vi "Sender UI.vi"(11 "error in (no error)":errorcluster) -> (15 "Error Out":errorcluster)   [LabVIEW 2022 SP3, in "Sender.lvclass"]
doc: "This VI acts as a sender where user selects the data type and the transmission type to send to the receiver."
uses:
  Sender.lvclass
  Controls/Operation.ctl
  Controls/State Cluster.ctl
  Controls/Sender Data Cluster.ctl
  Controls/Communication Mode.ctl
  Communication/Communication.lvclass
  Controls/User Event Operation.ctl
  Downloads/Sample PC Template/Sample PC Template/Typedefs/Data.ctl
  Downloads/Sample PC Template/Sample PC Template/Sample PC Template.lvlib
panel:
  in  "Stop Data":bool
  in  "Transmission Type":T1=enum."Notify With Data"
  in  "Data Type":string(combo)="Numeric Data"
  in  "Send":bool
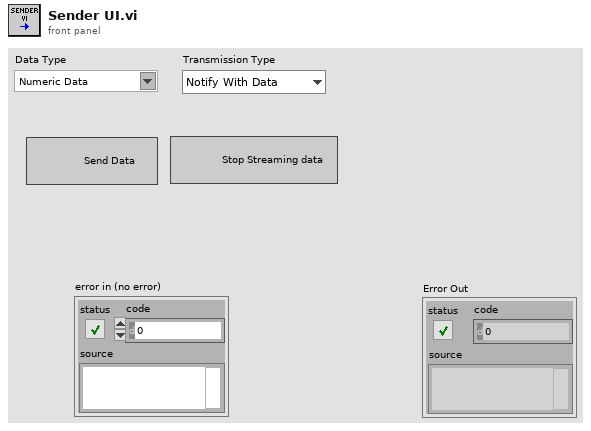
[diagram p1: front panel]
types:
  T1 = typedef "Communication Mode.ctl" = enum16{"Notify", "Notify With Data", "Stream Data"}
  T2 = typedef "User Event Operation.ctl" = enum16{"Obtain", "Generate", "Release"}
  T3 = typedef "State Cluster.ctl" = cluster{"State":string, "Data":variant}
  T4 = typedef "Operation.ctl" = enum16{"Create", "Enqueue", "Enqueue N", "Enstack", "Dequeue", "Flush", "Release"}
  T5 = enum8{"Enabled", "Disabled", "Disabled and Grayed Out"}
  T6 = typedef "Sample PC Template.lvlib/Data.ctl" = cluster{"State":string, "Data":variant}
  T7 = typedef "Sender Data Cluster.ctl" = cluster{"user event out":refnum<user-event>, "Selected Data Type":string, "Receiver VI Reference":refnum<vi>, "Transmission Type":T1, "Start Time":dbl, "Stop Stream Data":bool, "Communication Parent Class":refnum<class "Communication.lvclass">}
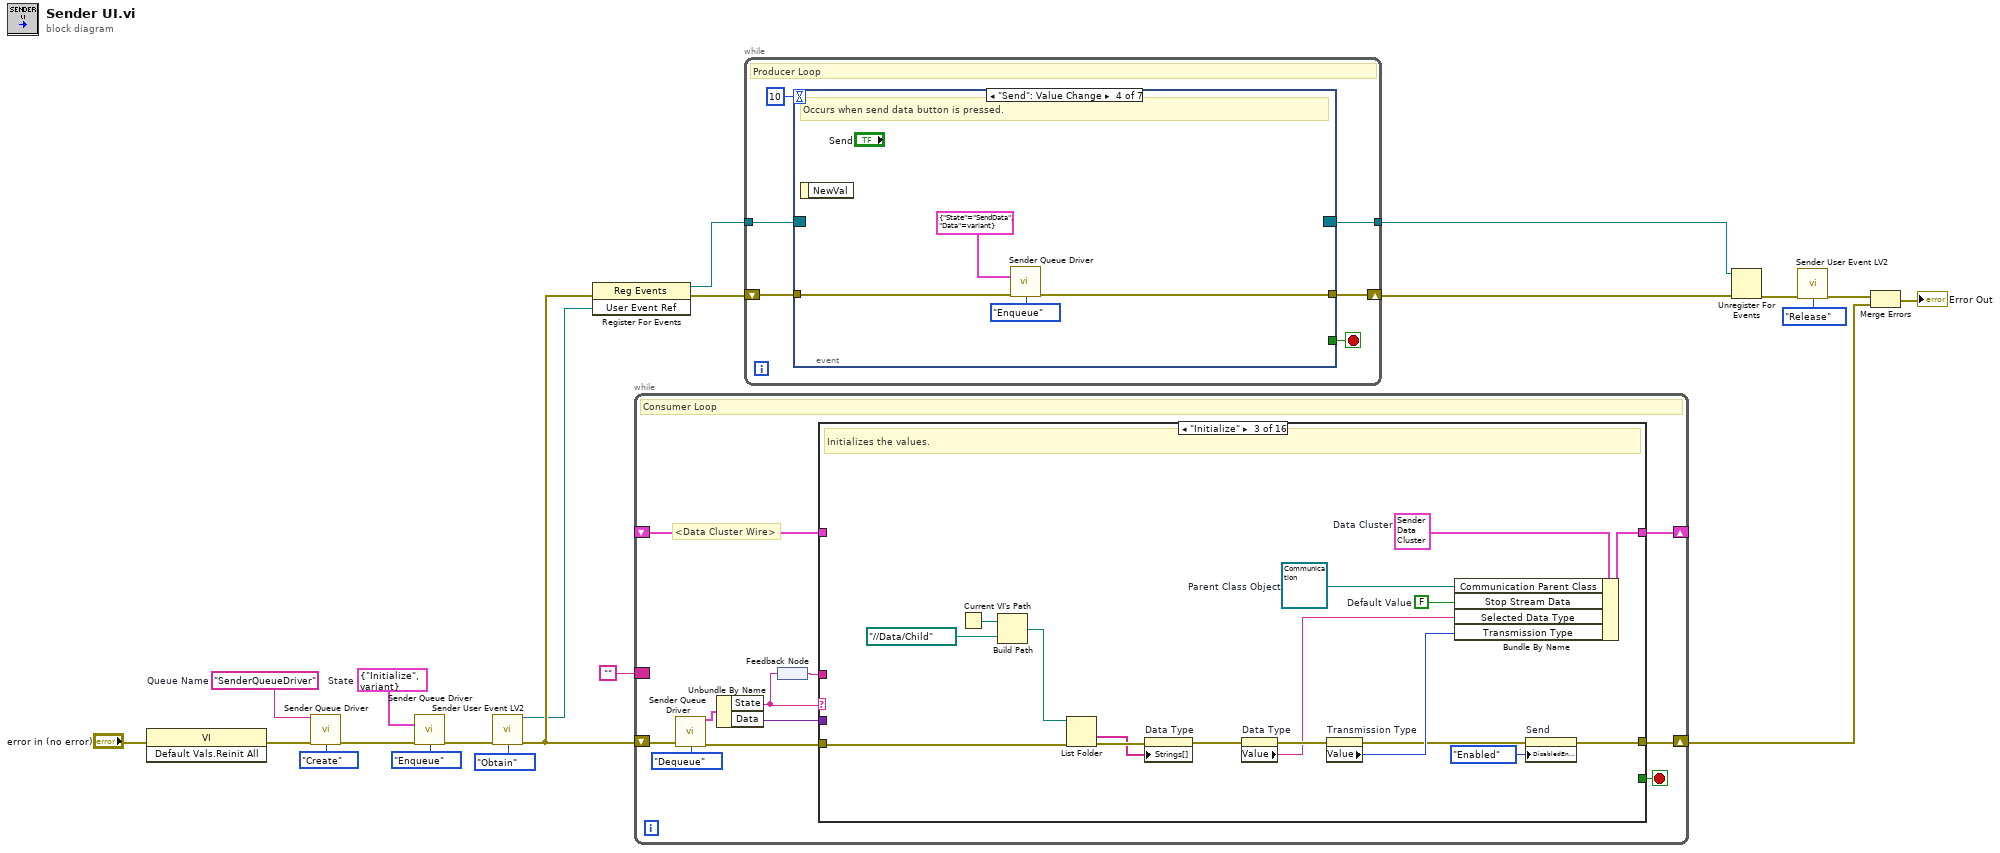
[diagram p0: block diagram]
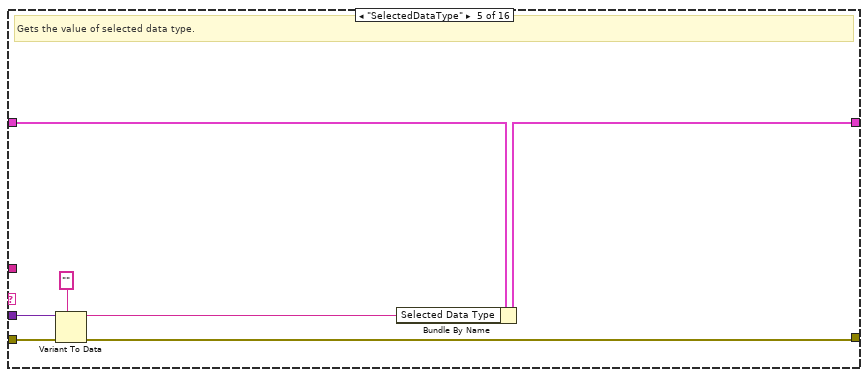
[diagram p5: hidden frame]
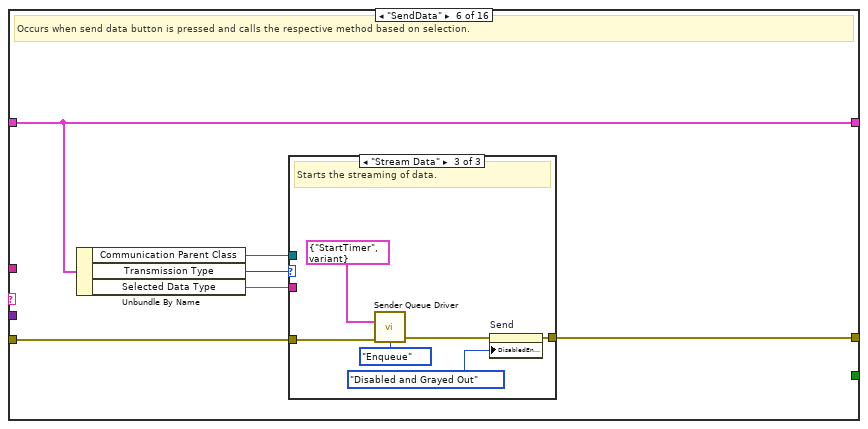
[diagram p6: hidden frame]
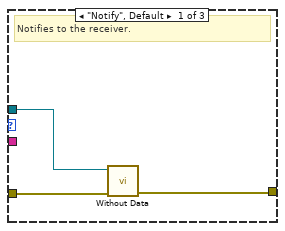
[diagram p7: hidden frame]
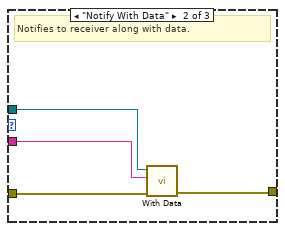
[diagram p8: hidden frame]
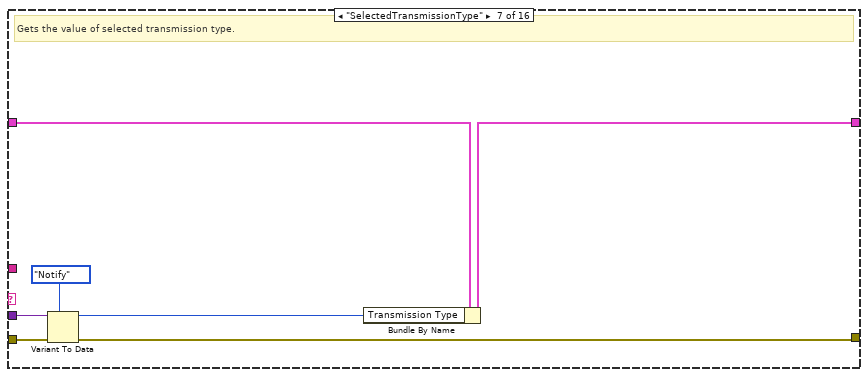
[diagram p9: hidden frame]
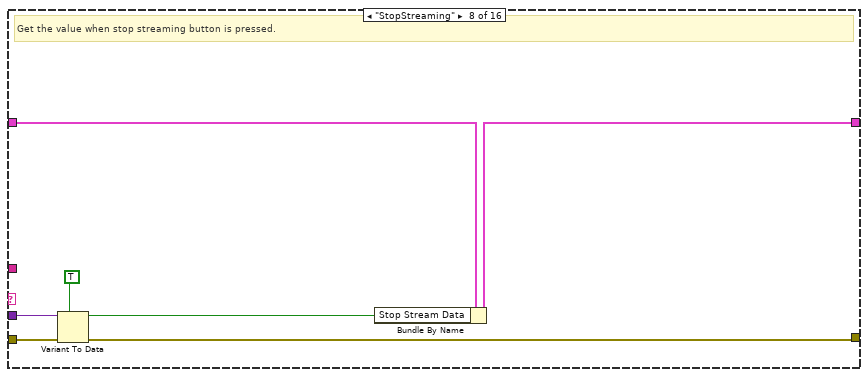
[diagram p10: hidden frame]
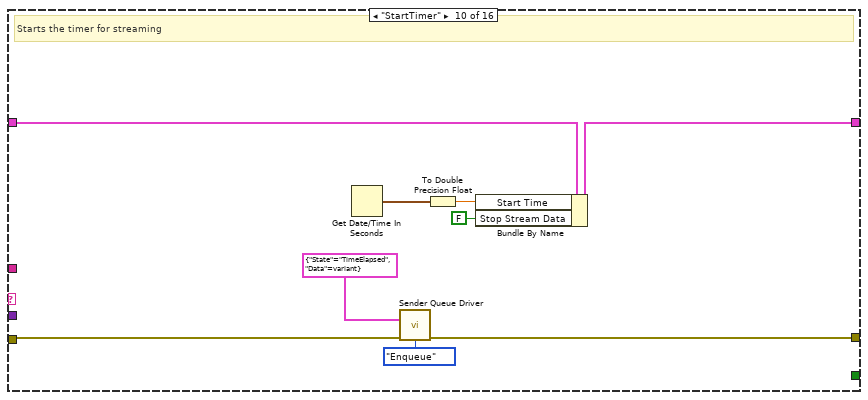
[diagram p12: hidden frame]
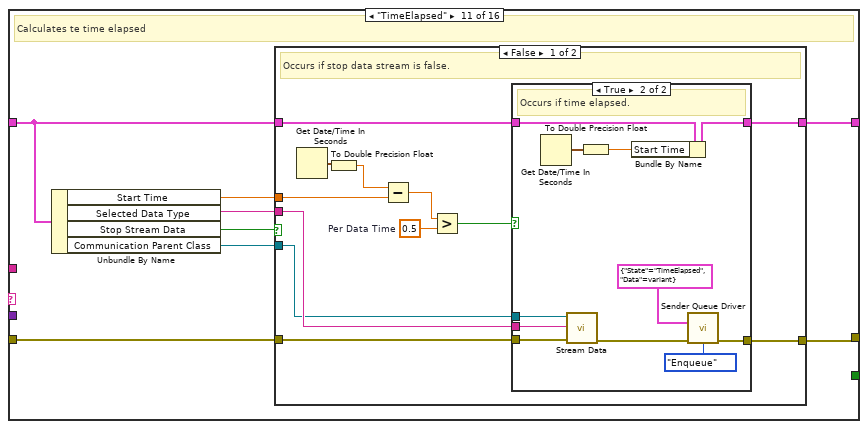
[diagram p13: hidden frame]
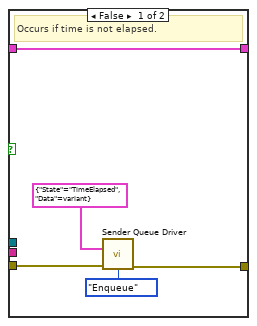
[diagram p14: hidden frame]
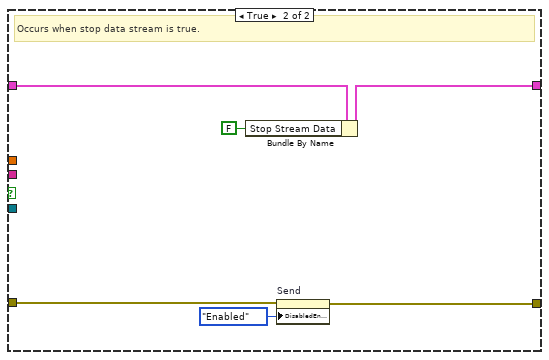
[diagram p15: hidden frame]
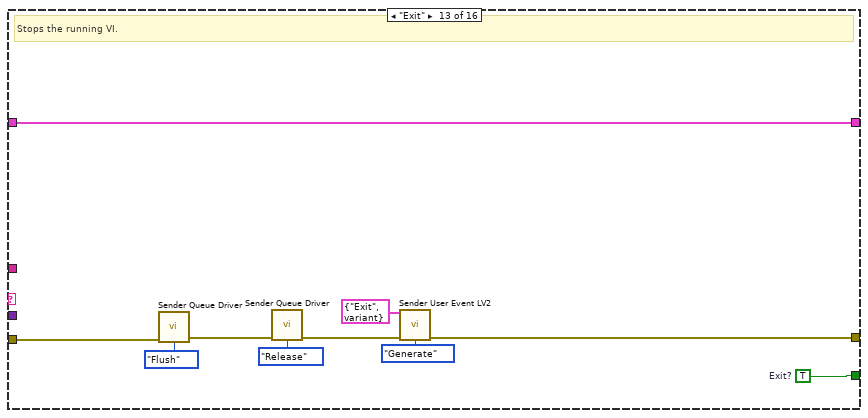
[diagram p17: hidden frame]
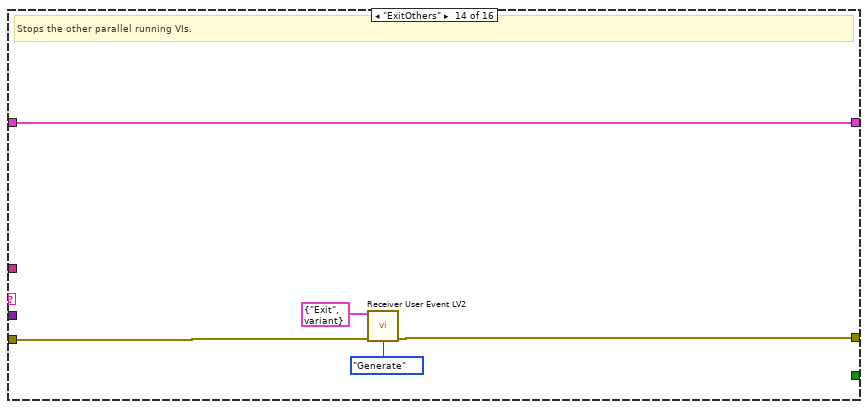
[diagram p18: hidden frame]
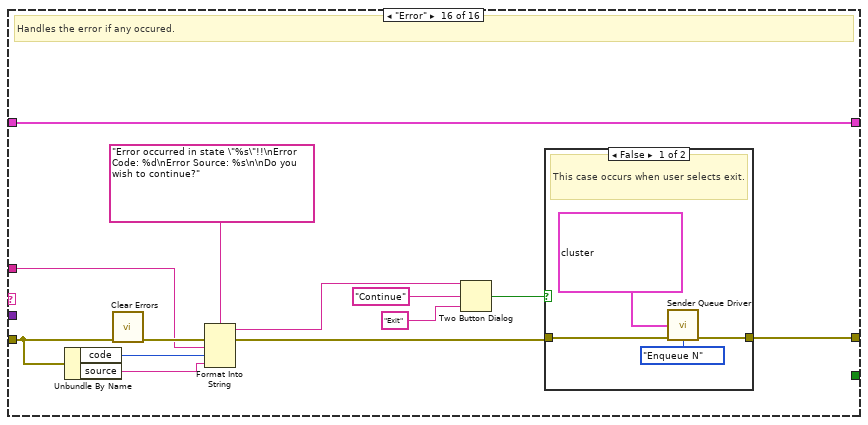
[diagram p20: hidden frame]
diagram:
  w15 = "SenderQueueDriver"  # Queue Name
  w17 = T3 {"State"="Initialize", "Data"=variant}  # State
  n1 = invoke class="VI" method="Default Vals.Reinit All"(error in="error in (no error)") -> (error out=w1:errorcluster)  [unwired: 2 in, 2 out]
  n2 = call "Sender Queue Driver.vi"("Queue Name"=w15, "error in (no error)"=w1, "Operations"=Operation."Create") -> ("error out"=w19:errorcluster)  [unwired: 11 in, 1 out]
  n3 = call "Sender Queue Driver.vi"("State"=w17, "error in (no error)"=w19, "Operations"=Operation."Enqueue") -> ("error out"=w8:errorcluster)  [unwired: 11 in, 1 out]
  n4 = call "Sender User Event LV2.vi"("Error In"=w8, "Operation"=User_Event_Operation."Obtain") -> ("User Event Ref"=w5:refnum<user-event>, "Error Out"=w7:errorcluster)  [unwired: 12 in]
  n5 = register-events(error in=w7, w5) -> (reference out=w13:refnum<event-registration>, error out=w14:errorcluster)  [unwired: 1 in]
  n6 = while {
    shift-right: [w25] -> w10
    shift-left: w7 -> [w31]
    border: "" -> [_]
    shift-right: [w22] -> _
    shift-left: _ -> [w23]
    stop <- w24 stop-if-true
    # "<Data Cluster Wire>"
    # "Consumer Loop"
    n7 = call "Sender Queue Driver.vi"("error in (no error)"=w31, "Operations"=Operation."Dequeue") -> ("Dequeued Element"=w30:T3, "error out"=w28:errorcluster)  [unwired: 12 in]
    n8 = Unbundle By Name(w30) -> ("State"=w27:string, "Data"=w29:variant)
    n9 = feedback-in #1(w27) -> ()
    n10 = feedback #1() -> (w26:string)
    n11 = case shown="\"Initialize\"" w27 {
      tunnel: w29 -> [_ _ _ _ w61 _ w86 w92 _ _ _ _ _ _ _ _]
      tunnel: w28 -> [w34 w36 w50 w55 w62 w68 w88 w95 w97 w102 w113 w150 w159 w164 w167 w173]
      tunnel: w26 -> [_ _ _ _ _ _ _ _ _ _ _ _ _ _ _ w169]
      tunnel: [w34 w36 w38 w55 w59 w67 w87 w94 w97 w101 w112 w150 w153 w163 w167 w172] -> w25
      tunnel: [_ _ _ _ _ _ _ _ _ _ _ _ w160 _ _ _] -> w24
      tunnel: w23 -> [w33 w35 _ w54 w58 w66 w84 w91 w96 w106 w110 w149 w155 w165 w166 w168]
      tunnel: [w33 w35 w53 w54 w57 w66 w82 w90 w96 w105 w109 w149 w155 w165 w166 w168] -> w22
      frame Default {
        # "Occurs if there is any developer error"
      }
      frame "/******** Initialization ********/" {
      }
      frame "Initialize" {
        w40 = refnum<class "Communication.lvclass"> refnum  # Parent Class Object
        w41 = T7 {"user event out"=refnum, "Selected Data Type"="", "Receiver VI Reference"=refnum, "Transmission Type"=enum."Notify", "Start Time"=0.0, "Stop Stream Data"=FALSE, "Communication Parent Class"=refnum}  # Data Cluster
        w46 = FALSE  # Default Value
        # "Initializes the values."
        n12 = Current VI's Path() -> (path=w52:path)
        n13 = Build Path(base path=w52, name or relative path=path "../../Data/Child") -> (appended path=w49:path)
        n14 = List Folder(path=w49, error in=w50) -> (folder names=w47:string[], error out=w48:errorcluster)  [unwired: 2 in, 2 out]
        n15 = property on="Data Type" class="CmbBox"(error in=w48, "Strings[]"=w47) -> (error out=w45:errorcluster)  [unwired: 1 in, 1 out]
        n16 = property on="Data Type" class="CmbBox"(error in=w45) -> (error out=w44:errorcluster, "Value"=w42:string)  [unwired: 1 in, 1 out]
        n17 = property on="Transmission Type" class="Enum (strict)"(error in=w44) -> (error out=w39:errorcluster, "Value"=w43:T1)  [unwired: 1 in, 1 out]
        n18 = Bundle By Name(cluster=w41, "Communication Parent Class"=w40, "Stop Stream Data"=w46, "Selected Data Type"=w42, "Transmission Type"=w43) -> (w53:T7)
        n19 = property on="Send" class="Bool"(error in=w39, "DisabledEnum"=T5."Enabled" ("Disabled")) -> (error out=w38:errorcluster)  [unwired: 1 in, 1 out]
      }
      frame "/********* Functionalities *********/" {
      }
      frame "SelectedDataType" {
        # "Gets the value of selected data type."
        n20 = Variant To Data(error in=w62, type="", Variant=w61) -> (data=w56:string, error out=w59:errorcluster)
        n21 = Bundle By Name(cluster=w58, "Selected Data Type"=w56) -> (w57:T7)
      }
      frame "SendData" {
        # "Occurs when send data button is pressed and calls the respective method based on selection."
        n22 = Unbundle By Name(w66) -> ("Communication Parent Class"=w63:refnum<class "Communication.lvclass">, "Transmission Type"=w65:T1, "Selected Data Type"=w64:string)
        n23 = case shown="\"Stream Data\"" w65 {
          tunnel: w68 -> [w71 w75 w81]
          tunnel: [w69 w74 w77] -> w67
          tunnel: w64 -> [_ w73 _]
          tunnel: w63 -> [w70 w72 _]
          frame "Notify", Default {
            # "Notifies to the receiver."
            n24 = call "Without Data.vi"("Error In"=w71, "Communication In"=w70) -> ("Error Out"=w69:errorcluster)  [unwired: 8 in, 1 out]
          }
          frame "Notify With Data" {
            # "Notifies to receiver along with data."
            n25 = call "With Data.vi"("Error In"=w75, "Data Type"=w73, "Communication In"=w72) -> ("Error Out"=w74:errorcluster)  [unwired: 7 in, 1 out]
          }
          frame "Stream Data" {
            # "Starts the streaming of data."
            n26 = call "Sender Queue Driver.vi"("State"=T3 {"State"="StartTimer", "Data"=variant}, "error in (no error)"=w81, "Operations"=Operation."Enqueue") -> ("error out"=w78:errorcluster)  [unwired: 11 in, 1 out]
            n27 = property on="Send" class="Bool"(error in=w78, "DisabledEnum"=T5."Disabled and Grayed Out" ("Disabled")) -> (error out=w77:errorcluster)  [unwired: 1 in, 1 out]
          }
        }
      }
      frame "SelectedTransmissionType" {
        # "Gets the value of selected transmission type."
        n28 = Variant To Data(error in=w88, type=Communication_Mode."Notify" ("Communication Mode"), Variant=w86) -> (data=w83:T1, error out=w87:errorcluster)
        n29 = Bundle By Name(cluster=w84, "Transmission Type"=w83) -> (w82:T7)
      }
      frame "StopStreaming" {
        # "Get the value when stop streaming button is pressed."
        n30 = Variant To Data(error in=w95, type=TRUE, Variant=w92) -> (data=w89:bool, error out=w94:errorcluster)
        n31 = Bundle By Name(cluster=w91, "Stop Stream Data"=w89) -> (w90:T7)
      }
      frame "/******* Timer Functionalities ********/" {
      }
      frame "StartTimer" {
        # "Starts the timer for streaming"
        n32 = Get Date/Time In Seconds() -> (seconds since 1Jan1904=w103:timestamp)
        n33 = call "Sender Queue Driver.vi"("State"=T3 {"State"="TimeElapsed", "Data"=variant}, "error in (no error)"=w102, "Operations"=Operation."Enqueue") -> ("error out"=w101:errorcluster)  [unwired: 11 in, 1 out]
        n34 = To Double Precision Float(number=w103) -> (double precision float=w104:dbl)
        n35 = Bundle By Name(cluster=w106, "Start Time"=w104, "Stop Stream Data"=FALSE) -> (w105:T7)
      }
      frame "TimeElapsed" {
        # "Calculates te time elapsed"
        n36 = Unbundle By Name(w110) -> ("Start Time"=w114:dbl, "Selected Data Type"=w111:string, "Stop Stream Data"=w108:bool, "Communication Parent Class"=w107:refnum<class "Communication.lvclass">)
        n37 = case shown="False" w108 {
          tunnel: w114 -> [w116 _]
          tunnel: w113 -> [w123 w145]
          tunnel: [w122 w144] -> w112
          tunnel: w111 -> [w120 _]
          tunnel: w110 -> [w119 w148]
          tunnel: [w118 w146] -> w109
          tunnel: w107 -> [w115 _]
          frame False {
            w124 = 0.5  # Per Data Time
            # "Occurs if stop data stream is false."
            n38 = Get Date/Time In Seconds() -> (seconds since 1Jan1904=w126:timestamp)
            n39 = To Double Precision Float(number=w126) -> (double precision float=w117:dbl)
            n40 = Subtract(x=w117, y=w116) -> (x-y=w125:dbl)
            n41 = Greater?(x=w125, y=w124) -> (0:w121:bool)
            n42 = case shown="True" w121 {
              tunnel: w123 -> [w131 w142]
              tunnel: [w130 w135] -> w122
              tunnel: w120 -> [_ w141]
              tunnel: w119 -> [w127 w140]
              tunnel: [w127 w139] -> w118
              tunnel: w115 -> [_ w132]
              frame False {
                # "Occurs if time is not elapsed."
                n43 = call "Sender Queue Driver.vi"("State"=T3 {"State"="TimeElapsed", "Data"=variant}, "error in (no error)"=w131, "Operations"=Operation."Enqueue") -> ("error out"=w130:errorcluster)  [unwired: 11 in, 1 out]
              }
              frame True {
                # "Occurs if time elapsed."
                n44 = Get Date/Time In Seconds() -> (seconds since 1Jan1904=w138:timestamp)
                n45 = call "Stream Data.vi"("Error In"=w142, "Data Type"=w141, "Communication In"=w132) -> ("Error Out"=w136:errorcluster)  [unwired: 7 in, 1 out]
                n46 = To Double Precision Float(number=w138) -> (double precision float=w137:dbl)
                n47 = Bundle By Name(cluster=w140, "Start Time"=w137) -> (w139:T7)
                n48 = call "Sender Queue Driver.vi"("State"=T3 {"State"="TimeElapsed", "Data"=variant}, "error in (no error)"=w136, "Operations"=Operation."Enqueue") -> ("error out"=w135:errorcluster)  [unwired: 11 in, 1 out]
              }
            }
          }
          frame True {
            # "Occurs when stop data stream is true."
            n49 = Bundle By Name(cluster=w148, "Stop Stream Data"=FALSE) -> (w146:T7)
            n50 = property on="Send" class="Bool"(error in=w145, "DisabledEnum"=T5."Enabled" ("Disabled")) -> (error out=w144:errorcluster)  [unwired: 1 in, 1 out]
          }
        }
      }
      frame "/******** Exit **********/" {
      }
      frame "Exit" {
        w160 = TRUE  # Exit?
        # "Stops the running VI."
        n51 = call "Sender Queue Driver.vi"("error in (no error)"=w159, "Operations"=Operation."Flush") -> ("error out"=w158:errorcluster)  [unwired: 12 in, 1 out]
        n52 = call "Sender Queue Driver.vi"("error in (no error)"=w158, "Operations"=Operation."Release") -> ("error out"=w154:errorcluster)  [unwired: 12 in, 1 out]
        n53 = call "Sender User Event LV2.vi"("Data"=T6 {"State"="Exit", "Data"=variant}, "Error In"=w154, "Operation"=User_Event_Operation."Generate") -> ("Error Out"=w153:errorcluster)  [unwired: 11 in, 1 out]
      }
      frame "ExitOthers" {
        # "Stops the other parallel running VIs."
        n54 = call "Receiver User Event LV2.vi"("Data"=T6 {"State"="Exit", "Data"=variant}, "Error In"=w164, "Operation"=User_Event_Operation."Generate") -> ("Error Out"=w163:errorcluster)  [unwired: 11 in, 1 out]
      }
      frame "/*********  Error Handling **********/" {
      }
      frame "Error" {
        # "Handles the error if any occured."
        n55 = Unbundle By Name(w173) -> ("code"=w171:i32, "source"=w170:string)
        n56 = call <vilib>:"Clear Errors.vi"("error in (no error)"=w173) -> ("error out"=w180:errorcluster)  [unwired: 5 in, 1 out]
        n57 = Format Into String(format string="Error occurred in state \"%s\"!!\nError Code: %d\nError Source: %s\n\nDo you wish to continue?", error in=w180, w169, w171, w170) -> (resulting string=w178:string, error out=w175:errorcluster)  [unwired: 1 in]
        n58 = Two Button Dialog(message=w178, 1:"Exit" ("F button name (\"Cancel\")"), 2:"Continue" ("T button name (\"OK\")")) -> (T button?=w174:bool)
        n59 = case shown="False" w174 {
          tunnel: w175 -> [w182 w185]
          tunnel: [w184 w185] -> w172
          frame False {
            # "This case occurs when user selects exit."
            n60 = call "Sender Queue Driver.vi"("State []"=T3[] [{"State"="ExitOthers", "Data"=variant}, {"State"="Exit", "Data"=variant}], "error in (no error)"=w182, "Operations"=Operation."Enqueue N") -> ("error out"=w184:errorcluster)  [unwired: 11 in, 1 out]
          }
          frame True {
            # "This case occurs when user selects to continue."
          }
        }
      }
    }
  }
  n61 = while {
    shift-right: [w188] -> w12
    shift-left: w14 -> [w189]
    tunnel: w13 -> [w190]
    tunnel: [w186] -> w11
    stop <- w187 stop-if-true
    # "Producer Loop"
    n62 = event shown="[3] \"Send\": Value Change" {
      selector: w190 -> [_ _ _ _ _ _ _]
      dyn-events: [_ _ _ _ _ _ _] -> w186
      timeout: 10 -> [_ _ _ _ _ _ _]
      tunnel: w189 -> [w192 w199 w206 w210 w217 w220 w232]
      tunnel: [w192 w198 w205 w209 w216 w218 w231] -> w188
      tunnel: [_ _ _ _ _ w219 _] -> w187
      event Timeout {
        # "This event occurs when no other event occurs"
        n63 = event-data() -> ()  [unwired: 1 in, 1 out]
      }
      event "Data Type": Value Change {
        # "Occurs when data type is selected by user."
        n64 = event-data() -> ("NewVal"=w194:string)  [unwired: 1 in]
        n65 = To Variant(anything=w194) -> (Variant=w195:variant)
        n66 = Bundle By Name(cluster=T3 {"State"="SelectedDataType", "Data"=variant} ("State"), "Data"=w195) -> (w193:T3)
        n67 = call "Sender Queue Driver.vi"("State"=w193, "error in (no error)"=w199, "Operations"=Operation."Enqueue") -> ("error out"=w198:errorcluster)  [unwired: 11 in, 1 out]
      }
      event Value Change {
        # "Occurs when communication mode is selected by user."
        n68 = event-data() -> ()  [unwired: 1 in, 1 out]
        n69 = To Variant(anything="Transmission Type") -> (Variant=w201:variant)
        n70 = Bundle By Name(cluster=T3 {"State"="SelectedTransmissionType", "Data"=variant} ("State"), "Data"=w201) -> (w200:T3)
        n71 = call "Sender Queue Driver.vi"("State"=w200, "error in (no error)"=w206, "Operations"=Operation."Enqueue") -> ("error out"=w205:errorcluster)  [unwired: 11 in, 1 out]
      }
      event "Send": Value Change {
        # "Occurs when send data button is pressed."
        n72 = event-data() -> ()  [unwired: 1 in, 1 out]
        n73 = call "Sender Queue Driver.vi"("State"=T3 {"State"="SendData", "Data"=variant}, "error in (no error)"=w210, "Operations"=Operation."Enqueue") -> ("error out"=w209:errorcluster)  [unwired: 11 in, 1 out]
      }
      event "Stop Data": Value Change {
        # "Occurs when stop streaming data is pressed."
        n74 = event-data() -> ()  [unwired: 1 in, 1 out]
        n75 = To Variant(anything=TRUE) -> (Variant=w213:variant)
        n76 = Bundle By Name(cluster=T3 {"State"="StopStreaming", "Data"=variant} ("State"), "Data"=w213) -> (w211:T3)
        n77 = call "Sender Queue Driver.vi"("State"=w211, "error in (no error)"=w217, "Operations"=Operation."Enqueue") -> ("error out"=w216:errorcluster)  [unwired: 11 in, 1 out]
      }
      event User Event {
        # "Occurs when this user event is generated."
        n78 = event-data() -> ("State"=w221:string)  [unwired: 1 in]
        n79 = case shown="\"Exit\"" w221 {
          tunnel: w220 -> [w222 w223 w228]
          tunnel: [_ w224 _] -> w219
          tunnel: [w222 w223 w227] -> w218
          frame Default {
          }
          frame "Exit" {
            w224 = TRUE  # Exit?
            # "Exists the producer loop."
          }
          frame "ExitConsumer" {
            # "Exists the consumer loop."
            n80 = call "Sender Queue Driver.vi"("State"=T3 {"State"="Exit", "Data"=variant}, "error in (no error)"=w228, "Operations"=Operation."Enqueue") -> ("error out"=w227:errorcluster)  [unwired: 11 in, 1 out]
          }
        }
      }
      event Panel Close? {
        w233 = TRUE  # Discard?
        # "Occurs when panel close is pressed"
        n81 = event-data() -> ()  [unwired: 1 in, 1 out]
        n82 = call "Sender Queue Driver.vi"("State []"=T3[] [{"State"="ExitOthers", "Data"=variant}, {"State"="Exit", "Data"=variant}], "error in (no error)"=w232, "Operations"=Operation."Enqueue N") -> ("error out"=w231:errorcluster)  [unwired: 11 in, 1 out]
        n83 = event-data("Discard?"=w233) -> ()  [unwired: 1 in, 1 out]
      }
    }
  }
  n84 = Unregister For Events(event registration refnum=w11, error in=w12) -> (error out=w4:errorcluster)
  n85 = call "Sender User Event LV2.vi"("Error In"=w4, "Operation"=User_Event_Operation."Release") -> ("Error Out"=w3:errorcluster)  [unwired: 12 in, 1 out]
  n86 = Merge Errors(w3, w10) -> (→"Error Out":errorcluster)
